vi "Timer IRQ Config Pane.vi"(6 "_SubPanelMessages":refnum<notifier>, 9 "_myEmbeddedToFrameEvent":T7, 10 "_myEmbedded.Exit":refnum<user-event>, 11 "_Property Bundle":cluster{"Name":string, "Value":variant}[](array[cluster])) -> (1 "_Connection Informations":T2, 2 "_Scripter Input":T4)   [LabVIEW 2021]
doc: "Registers analog and digital input interrupts and creates timer interrupts."
uses:
  <vilib>/myRIO/Common/Express VI Framework/typedefs/Config Pane to Framework Ref.ctl
  <vilib>/myRIO/Common/Express VI Framework/typedefs/Data Validate Ref.ctl
  <vilib>/myRIO/Common/Express VI Framework/typedefs/Sub Panel Messages.ctl
  <vilib>/myRIO/Common/Express VI Framework/typedefs/Instrument Driver Method Descriptor Array.ctl
  <vilib>/myRIO/Common/Express VI Framework/typedefs/Instrument Driver Method Descriptor.ctl
  <vilib>/myRIO/Common/Express VI Framework/typedefs/Scripter Input.ctl
  <vilib>/myRIO/Common/Express VI Framework/typedefs/WireThrough Terminal Names.ctl
  <vilib>/myRIO/Common/Express VI Framework/typedefs/Connection Informations.ctl
  <vilib>/myRIO/Common/Express VI Framework/vis/Express VI Framework Strings Global.vi
  <vilib>/myRIO/Express VI/IRQ/Message Globals.vi
panel:
  out "_create Callback?":bool
  in  "_Create Button":bool
  in  "Callback VI Path:":path
  out "_Warning Icon":picture
  out "_Callback VI Path":string caption="Callback VI:"
  in  "_Open Button":bool
  out "_Interval 2":string
  out "_Interval 1":string
  out "_Timer Preview":T1(graph) caption="Preview:"
  out "_Error Message":string
  in  "_callback":refnum<vi>
  in  "_VI Default Name (Edit and make value default)":string="Timer interrupt"
  in  "_WireThrough Info (Edit and make value default)":T3={"WireThrough Top In"="Ref In", "WireThrough Bottom In"="error in (no error)", "WireThrough Top Out"="Ref Out", "WireThrough Bottom Out"="error out"}
  in  "_Template Array (Edit and make value default)":T5=[{"Function Name"="Create Timer IRQ", "VI Path"=path "<vilib>/myRIO/Instrument Drivers/IRQ/Timer IRQ/vis", "Script"=TRUE, "Inputs"=[{"name"="Timer ID", "value"=variant, "Config Pane Only"=TRUE, "Build Array"=FALSE, "Bundle Cluster"=FALSE, "Show Term"=FALSE, "alias"=[], "Required Input"=FALSE}, {"name"="Interval [us]", "value"=variant, "Config Pane Only"=TRUE, "Build Array"=FALSE, "Bundle Cluster"=FALSE, "Show Term"=FALSE, "alias"=[], "Required Input"=FALSE}, {"name"="Callback VI Reference", "value"=variant, "Config Pane Only"=FALSE, "Build Array"=FALSE, "Bundle Cluster"=FALSE, "Show Term"=TRUE, "alias"=[], "Required Input"=FALSE}], "Outputs"=[], "VI Class"=enum."Open", "Controls Refs[]"=[], "Inline"=FALSE}]
  in  "_Default Alias String":string
  in  "Timer ID:":u8 max=7
  in  "Interval (us):":u32=1000000 min=1
  in  "Name:":string="Timer interrupt" caption="Node name:"
  out "_IRQ Learn More":string="Interrupt triggers every time the specified Interval elapses."
  # "NOTE: Tab Order has been set\nfor this Front Panel.\n\nSee Edit>>Set Tabbing Order...\n\nAll controls that are not visible at \nruntime are excluded from Tabbing order\n\nTo exlude a control from context\nhelp prefix its label text with a '-'"
  # "Trigger point"
  # "Time"
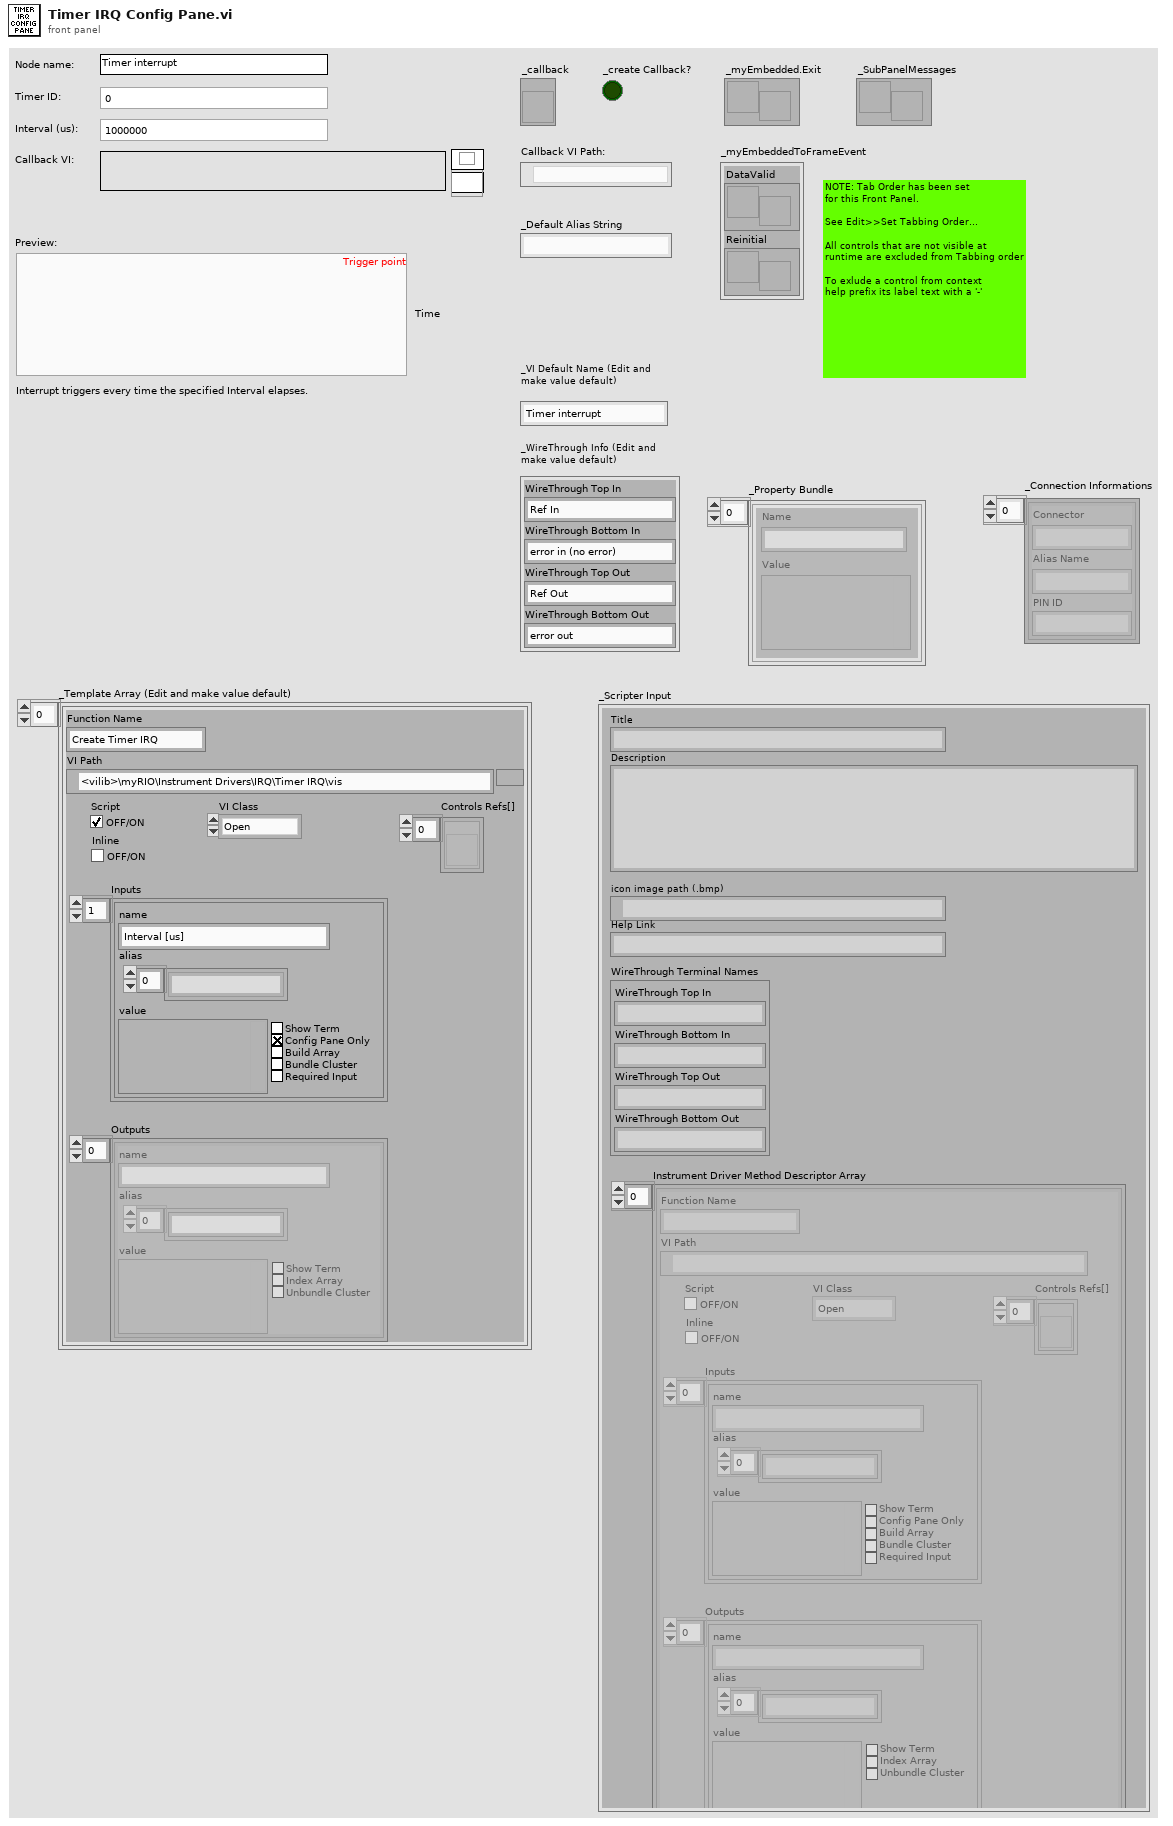
[diagram p1: front panel]
types:
  T1 = cluster{"Analog Preview 3":cluster{"X":sgl, "Y":sgl}[]}[]
  T2 = typedef "Connection Informations.ctl" = cluster{"Connector":string, "Alias Name":string, "PIN ID":string}[]
  T3 = typedef "WireThrough Terminal Names.ctl" = cluster{"WireThrough Top In":string, "WireThrough Bottom In":string, "WireThrough Top Out":string, "WireThrough Bottom Out":string}
  T4 = typedef "Scripter Input.ctl" = cluster{"Title":string, "Description":string, "icon image path (.bmp)":path, "Help Link":string, "WireThrough Terminal Names":T3, "Instrument Driver Method Descriptor Array":T5}
  T5 = typedef "Instrument Driver Method Descriptor Array.ctl" = T6[]
  T6 = typedef "Instrument Driver Method Descriptor.ctl" = cluster{"Function Name":string, "VI Path":path, "Script":bool, "Inputs":cluster{"name":string, "value":variant, "Config Pane Only":bool, "Build Array":bool, "Bundle Cluster":bool, "Show Term":bool, "alias":string[], "Required Input":bool}[], "Outputs":cluster{"name":string, "value":variant, "Show Term":bool, "Index Array":bool, "Unbundle Cluster":bool, "alias":string[]}[], "VI Class":enum16{"Open", "Configure", "Data", "Manage", "Close"}, "Controls Refs[]":refnum<vi>[], "Inline":bool}
  T7 = typedef "Config Pane to Framework Ref.ctl" = cluster{"DataValid":T8, "Reinitial":refnum<user-event>}
  T8 = typedef "Data Validate Ref.ctl" = refnum<user-event>
  T9 = typedef "Sub Panel Messages.ctl" = enum16{"Initialized"}
  T10 = cluster{"left":i16, "top":i16, "right":i16, "bottom":i16}
  T11 = cluster{"name":string, "value":variant, "Config Pane Only":bool, "Build Array":bool, "Bundle Cluster":bool, "Show Term":bool, "alias":string[], "Required Input":bool}[]
  T12 = cluster{"name":string, "value":variant, "Config Pane Only":bool, "Build Array":bool, "Bundle Cluster":bool, "Show Term":bool, "alias":string[], "Required Input":bool}
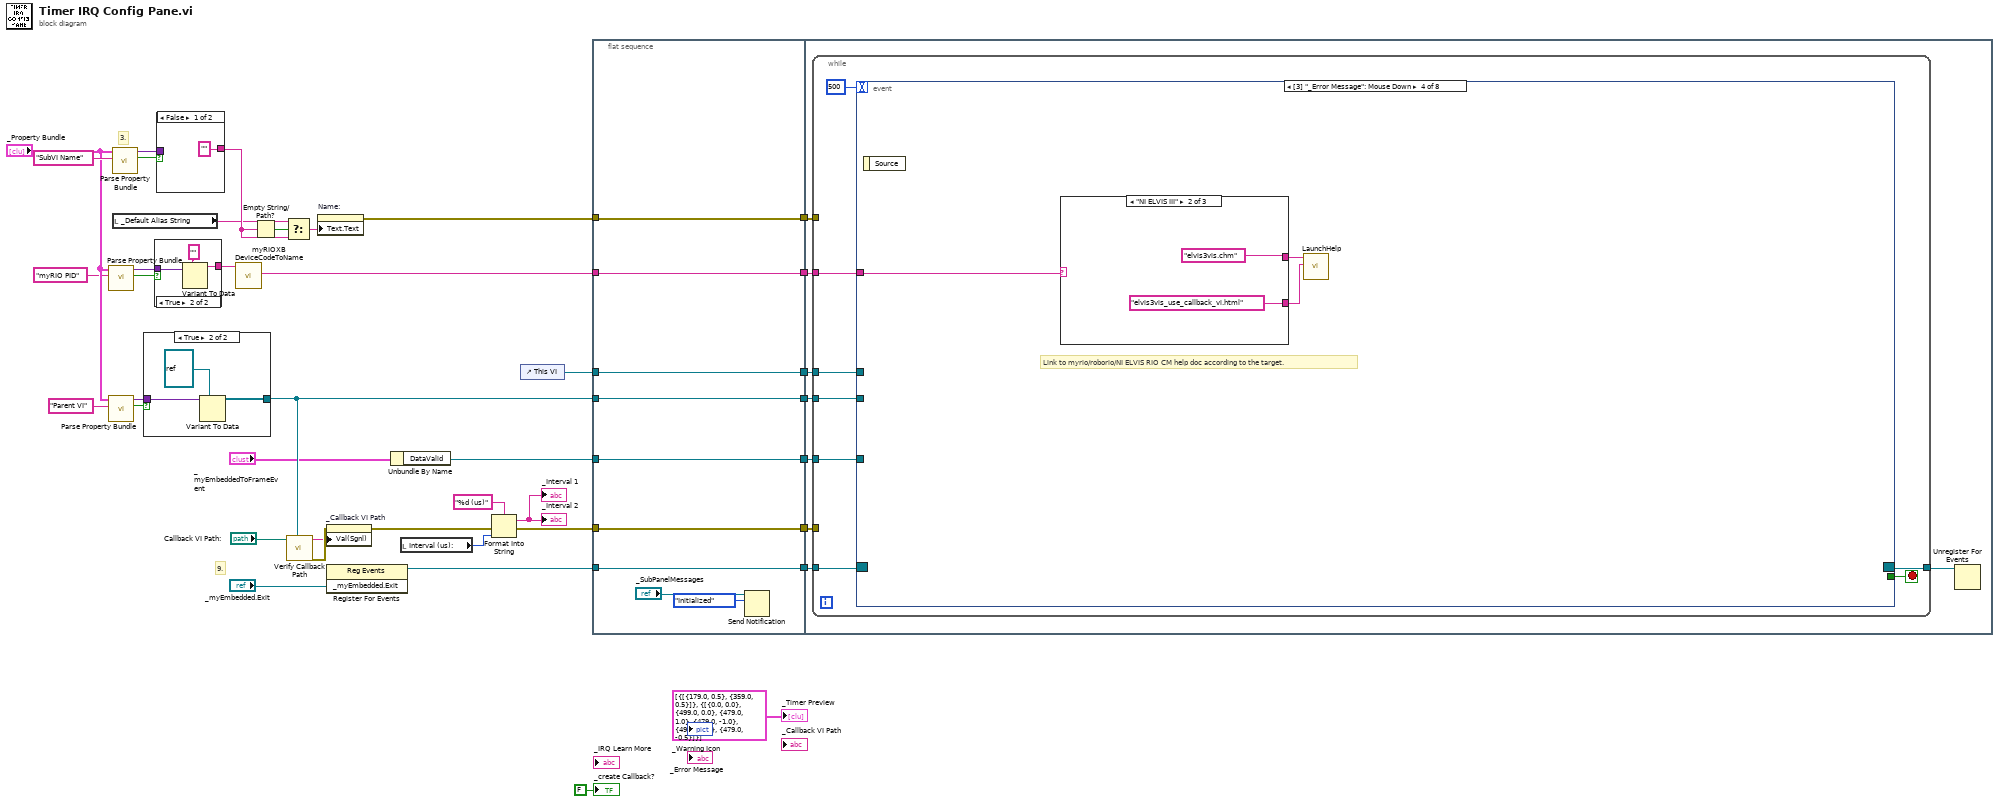
[diagram p0: block diagram]
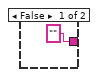
[diagram p2: hidden frame]
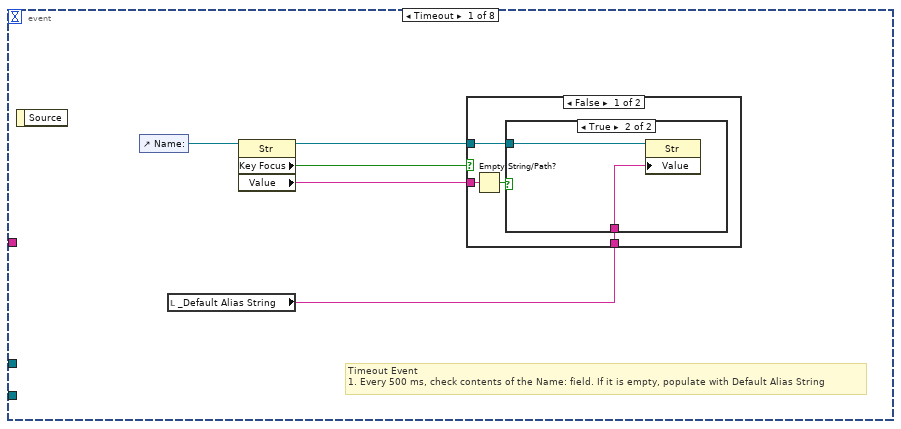
[diagram p3: hidden frame]
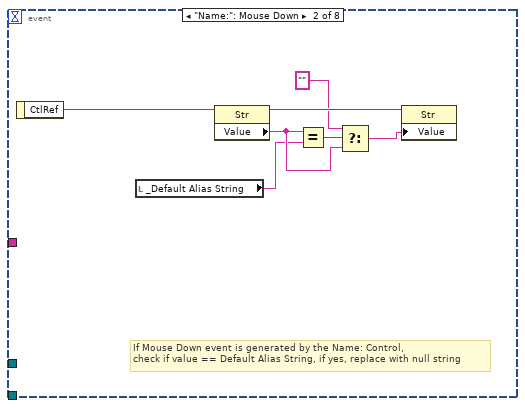
[diagram p6: hidden frame]
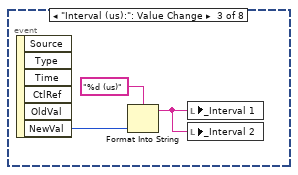
[diagram p7: hidden frame]
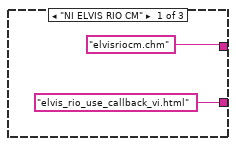
[diagram p8: hidden frame]
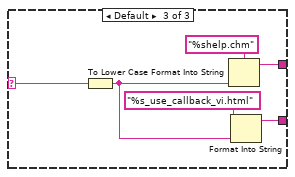
[diagram p9: hidden frame]
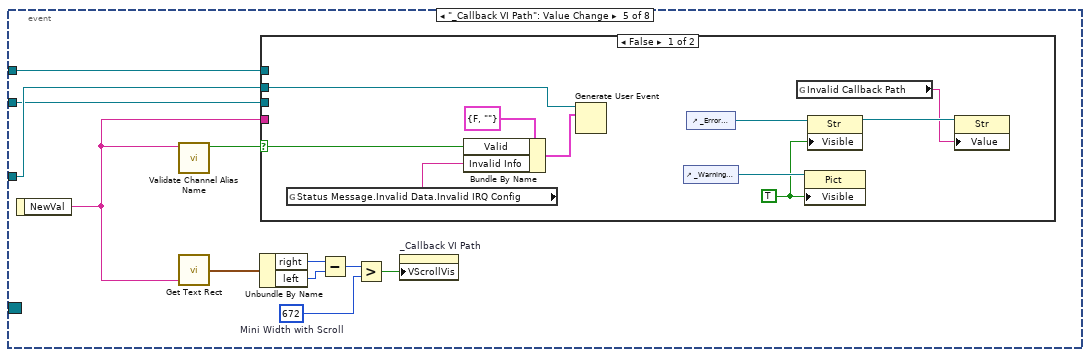
[diagram p10: hidden frame]
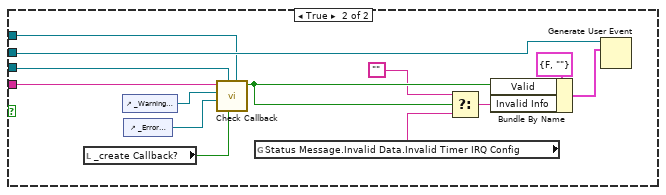
[diagram p11: hidden frame]
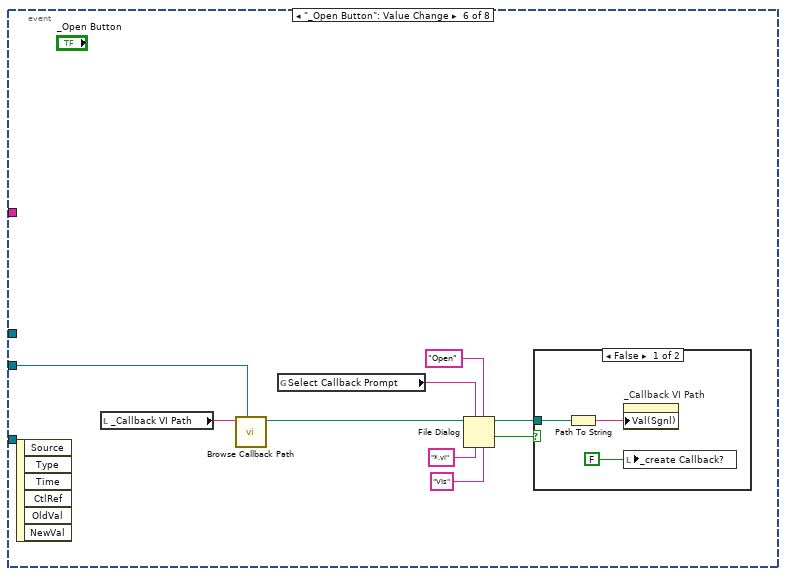
[diagram p12: hidden frame]
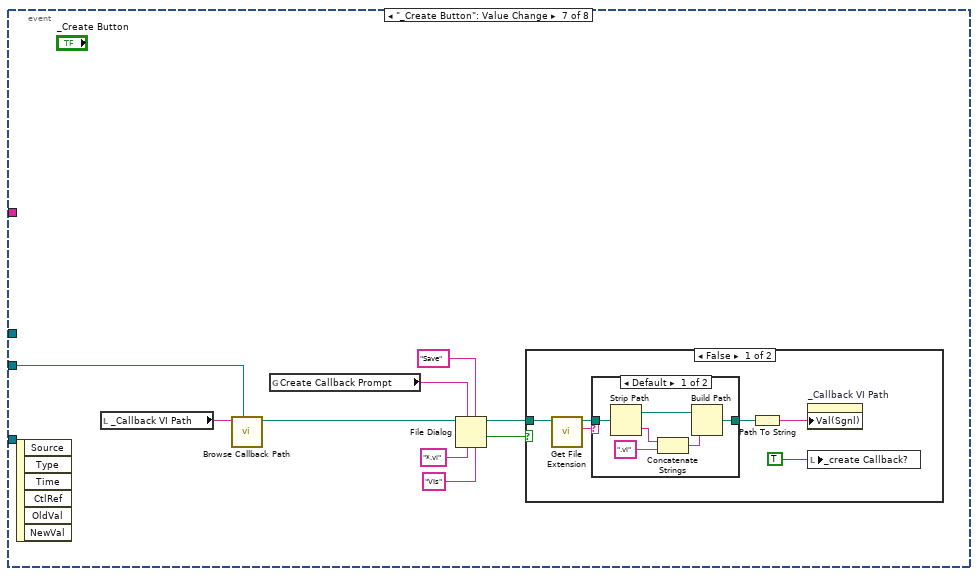
[diagram p14: hidden frame]
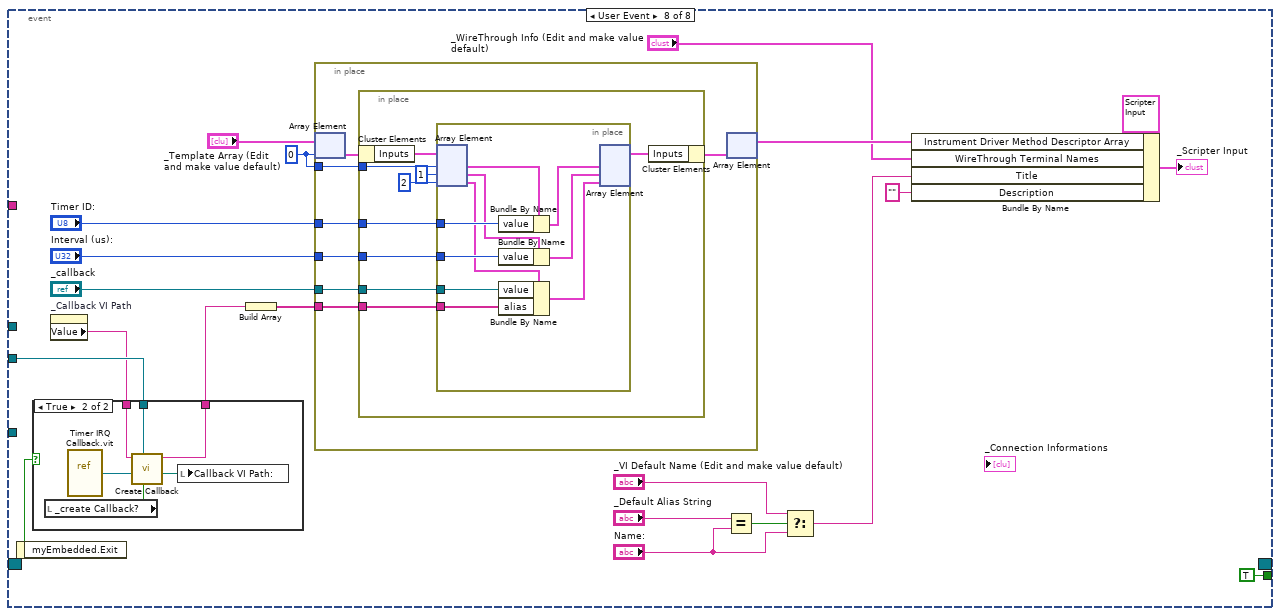
[diagram p17: hidden frame]
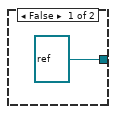
[diagram p19: hidden frame]
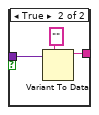
[diagram p20: hidden frame]
diagram:
  # "9."
  # "3."
  n1 = call <vilib>:"Parse Property Bundle.vi"("Name"="myRIO PID", "Property Bundle"="_Property Bundle") -> ("Found?"=w4:bool, "Value"=w5:variant)  [unwired: 8 in]
  n2 = call <vilib>:"Parse Property Bundle.vi"("Name"="Parent VI", "Property Bundle"="_Property Bundle") -> ("Found?"=w28:bool, "Value"=w29:variant)  [unwired: 8 in]
  n3 = call <vilib>:"Parse Property Bundle.vi"("Name"="SubVI Name", "Property Bundle"="_Property Bundle") -> ("Found?"=w37:bool, "Value"=w36:variant)  [unwired: 8 in]
  n4 = local read "_Default Alias String"() -> (w32:string)
  n5 = case shown="True" w28 {
    tunnel: w29 -> [_ w44]
    tunnel: [refnum<vi> refnum ("reference out") w42] -> w20
    frame False {
    }
    frame True {
      n6 = Variant To Data(type=refnum<vi> refnum ("reference out"), Variant=w44) -> (data=w42:refnum<vi>)  [unwired: 1 in, 1 out]
    }
  }
  n7 = case shown="True" w4 {
    tunnel: w5 -> [_ w48]
    tunnel: ["" ("Name") w46] -> w1
    frame False {
    }
    frame True {
      n8 = Variant To Data(type="" ("Name"), Variant=w48) -> (data=w46:string)  [unwired: 1 in, 1 out]
    }
  }
  n9 = case shown="False" w37 {
    tunnel: w36 -> [_ w52]
    tunnel: ["" ("Name") w50] -> w35
    frame False {
    }
    frame True {
      n10 = Variant To Data(type="" ("Name"), Variant=w52) -> (data=w50:string)  [unwired: 1 in, 1 out]
    }
  }
  n11 = call <vilib>:"myRIOXB DeviceCodeToName.vi"("Device Code"=w1) -> ("Name"=w2:string)  [unwired: 10 in]
  n12 = Empty String/Path?(string/path=w35) -> (empty?=w39:bool)
  n13 = Select(t=w32, s=w39, f=w35) -> (s? t:f=w31:string)
  n14 = call <vilib>:"Verify Callback Path.vi"("Parent VI Ref"=w20, "Saved Callback Path"="Callback VI Path:") -> ("error out"=w23:errorcluster, "Valid Path out"=w21:string)  [unwired: 8 in]
  n15 = property on="Name:" class="Str"("Text.Text"=w31) -> (error out=w33:errorcluster)  [unwired: 2 in, 1 out]
  n16 = property on="_Callback VI Path" class="Str"(error in=w23, "Val(Sgnl)"=w21) -> (error out=w22:errorcluster)  [unwired: 1 in, 1 out]
  n17 = register-events("_myEmbedded.Exit") -> (reference out=w34:refnum<event-registration>)  [unwired: 2 in, 1 out]
  n18 = Unbundle By Name("_myEmbeddedToFrameEvent") -> ("DataValid"=w15:T8)
  n19 = local read "Interval (us):"() -> (w25:u32)
  n20 = Format Into String(format string="%d (us)", error in=w22, w25) -> (resulting string=→"_Interval 1" →"_Interval 2":string, error out=w17:errorcluster)  [unwired: 1 in]
  n21 = control-ref of="This VI"() -> (w19:refnum<vi>)
  n22 = flat-sequence {
    tunnel: w15 -> [w56]
    tunnel: w17 -> [w57]
    tunnel: w19 -> [w58]
    tunnel: w20 -> [w59]
    tunnel: w33 -> [w60]
    tunnel: w34 -> [w61]
    tunnel: [w61] -> w14
    tunnel: [w60] -> w13
    tunnel: [w59] -> w12
    tunnel: [w58] -> w11
    tunnel: [w57] -> w10
    tunnel: [w56] -> w9
    tunnel: [w53] -> w3
    tunnel: w2 -> [w53]
    tunnel: w14 -> [w69]
    tunnel: w13 -> [w67]
    tunnel: w12 -> [w66]
    tunnel: w11 -> [w65]
    tunnel: w10 -> [w64]
    tunnel: w9 -> [w63]
    tunnel: w3 -> [w62]
    frame #0 {
      n23 = Send Notification(notification=Sub_Panel_Messages."Initialized", notifier="_SubPanelMessages") -> ()  [unwired: 1 in, 2 out]
    }
    frame #1 {
      n24 = while {
        tunnel: w69 -> [w76]
        tunnel: w63 -> [w73]
        tunnel: [w74] -> w68
        tunnel: w67 -> [_]
        tunnel: w66 -> [w72]
        tunnel: w65 -> [w71]
        tunnel: w64 -> [_]
        tunnel: w62 -> [w70]
        stop <- w75 stop-if-true
        n25 = event shown="[3] \"_Error Message\": Mouse Down" {
          selector: w76 -> [_ _ _ _ _ _ _ _]
          dyn-events: [_ _ _ _ _ _ _ _] -> w74
          timeout: 500 -> [_ _ _ _ _ _ _ _]
          tunnel: [_ _ _ _ _ _ _ TRUE ("Valid Callback?")] -> w75
          tunnel: w73 -> [_ _ _ _ w122 _ _ _]
          tunnel: w72 -> [_ _ _ _ w121 w147 w158 w184]
          tunnel: w71 -> [_ _ _ _ w120 _ _ _]
          tunnel: w70 -> [_ _ _ w99 _ _ _ _]
          event Timeout {
            # "Timeout Event\n1. Every 500 ms, check contents of the Name: field. If it is empty, populate with Default Alias String"
            n26 = event-data() -> ()  [unwired: 1 in, 1 out]
            n27 = control-ref of="Name:"() -> (w79:refnum<vi>)
            n28 = local read "_Default Alias String"() -> (w78:string)
            n29 = property on="Property Node" class="Str"(reference=w79) -> (reference out=w82:refnum<vi>, "Key Focus"=w81:bool, "Value"=w80:string)  [unwired: 1 in, 1 out]
            n30 = case shown="False" w81 {
              tunnel: w80 -> [w86 _]
              tunnel: w82 -> [w84 _]
              tunnel: w78 -> [w83 _]
              frame False {
                n31 = Empty String/Path?(string/path=w86) -> (empty?=w85:bool)
                n32 = case shown="True" w85 {
                  tunnel: w84 -> [_ w88]
                  tunnel: w83 -> [_ w87]
                  frame False {
                  }
                  frame True {
                    n33 = property on="Property Node" class="Str"(reference=w88, "Value"=w87) -> ()  [unwired: 1 in, 2 out]
                  }
                }
              }
              frame True {
              }
            }
          }
          event "Name:": Mouse Down {
            # "If Mouse Down event is generated by the Name: Control,\ncheck if value == Default Alias String, if yes, replace with null string"
            n34 = event-data() -> ("CtlRef"=w90:refnum<vi>)  [unwired: 1 in]
            n35 = local read "_Default Alias String"() -> (w89:string)
            n36 = property class="Str"(reference=w90) -> (reference out=w94:refnum<vi>, "Value"=w95:string)  [unwired: 1 in, 1 out]
            n37 = Equal?(x=w95, y=w89) -> (x = y?=w91:bool)
            n38 = Select(t="", s=w91, f=w95) -> (s? t:f=w93:string)
            n39 = property class="Str"(reference=w94, "Value"=w93) -> ()  [unwired: 1 in, 2 out]
          }
          event "Interval (us):": Value Change {
            n40 = event-data() -> ("NewVal"=w98:u32)  [unwired: 1 in, 5 out]
            n41 = Format Into String(format string="%d (us)", w98) -> (resulting string=w96:string)  [unwired: 2 in, 1 out]
            n42 = local write "_Interval 1"(w96) -> ()
            n43 = local write "_Interval 2"(w96) -> ()
          }
          event "_Error Message": Mouse Down {
            # "Link to myrio/roborio/NI ELVIS RIO CM help doc according to the target."
            n44 = event-data() -> ()  [unwired: 1 in, 1 out]
            n45 = case shown="\"NI ELVIS III\"" w99 {
              selector: w99 -> [_ _ w106]
              tunnel: ["elvisriocm.chm" ("Help File") "elvis3vis.chm" ("Help File") w108] -> w101
              tunnel: ["elvis_rio_use_callback_vi.html" ("Help Topic") "elvis3vis_use_callback_vi.html" ("Help Topic") w107] -> w100
              frame "NI ELVIS RIO CM" {
              }
              frame "NI ELVIS III" {
              }
              frame Default {
                n46 = To Lower Case(string=w106) -> (all lower case string=w110:string)
                n47 = Format Into String(format string="%shelp.chm" ("Help File"), w110) -> (resulting string=w108:string)  [unwired: 2 in, 1 out]
                n48 = Format Into String(format string="%s_use_callback_vi.html" ("Help Topic"), w110) -> (resulting string=w107:string)  [unwired: 2 in, 1 out]
              }
            }
            n49 = call <vilib>:"LaunchHelp.vi"("Help Topic"=w100, "Help File"=w101) -> ()  [unwired: 10 in]
          }
          event "_Callback VI Path": Value Change {
            w115 = i16 672  # Mini Width with Scroll
            n50 = event-data() -> ("NewVal"=w112:string)  [unwired: 1 in]
            n51 = call <vilib>:"Validate Channel Alias Name.vi"("Channel Alias"=w112) -> ("Valid?"=w113:bool)  [unwired: 9 in, 1 out]
            n52 = call <vilib>:"Get Text Rect.vi"("text"=w112) -> ("rect"=w119:T10)  [unwired: 8 in]
            n53 = Unbundle By Name(w119) -> ("right"=w118:i16, "left"=w117:i16)
            n54 = case shown="False" w113 {
              selector: w113 -> [w129 _]
              tunnel: w122 -> [w130 w145]
              tunnel: w121 -> [_ w144]
              tunnel: w120 -> [_ w141]
              tunnel: w112 -> [_ w140]
              frame False {
                w126 = TRUE ("Visible")
                n55 = global read "Express VI Framework Strings Global.vi" "Status Message.Invalid Data.Invalid IRQ Config"() -> (w125:string)
                n56 = Bundle By Name(cluster=cluster{"Valid":bool, "Invalid Info":string} {"Valid"=FALSE, "Invalid Info"=""} ("event data"), "Valid"=w129, "Invalid Info"=w125) -> (w131:cluster{"Valid":bool, "Invalid Info":string})
                n57 = Generate User Event(user event=w130, event data cluster=w131) -> ()  [unwired: 2 in, 2 out]
                n58 = control-ref of="_Warning Icon"() -> (w127:refnum<vi>)
                n59 = control-ref of="_Error Message"() -> (w128:refnum<vi>)
                n60 = global read "Message Globals.vi" "Invalid Callback Path"() -> (w123:string)
                n61 = property class="Pict"(reference=w127, "Visible"=w126) -> ()  [unwired: 1 in, 2 out]
                n62 = property class="Str"(reference=w128, "Visible"=w126) -> (reference out=w124:refnum<vi>)  [unwired: 1 in, 1 out]
                n63 = property class="Str"(reference=w124, "Value"=w123) -> ()  [unwired: 1 in, 2 out]
              }
              frame True {
                n64 = local read "_create Callback?"() -> (w139:bool)
                n65 = control-ref of="_Warning Icon"() -> (w142:refnum<vi>)
                n66 = control-ref of="_Error Message"() -> (w143:refnum<vi>)
                n67 = call <vilib>:"Check Callback.vi"("Config VI Ref"=w141, "Create Callback?"=w139, "Parent VI Ref"=w144, "Error Message Ref"=w143, "Warning Icon Ref"=w142, "Callback Path"=w140) -> ("Valid Callback?"=w136:bool)  [unwired: 5 in]
                n68 = global read "Express VI Framework Strings Global.vi" "Status Message.Invalid Data.Invalid Timer IRQ Config"() -> (w134:string)
                n69 = Select(t="", s=w136, f=w134) -> (s? t:f=w133:string)
                n70 = Bundle By Name(cluster=cluster{"Valid":bool, "Invalid Info":string} {"Valid"=FALSE, "Invalid Info"=""} ("event data"), "Valid"=w136, "Invalid Info"=w133) -> (w137:cluster{"Valid":bool, "Invalid Info":string})
                n71 = Generate User Event(user event=w145, event data cluster=w137) -> ()  [unwired: 2 in, 2 out]
              }
            }
            n72 = Subtract(x=w118, y=w117) -> (x-y=w116:i16)
            n73 = Greater?(x=w116, y=w115) -> (0:w114:bool)
            n74 = property on="_Callback VI Path" class="Str"("VScrollVis"=w114) -> ()  [unwired: 2 in, 2 out]
          }
          event "_Open Button": Value Change {
            n75 = event-data() -> ()  [unwired: 1 in, 6 out]
            n76 = local read "_Callback VI Path"() -> (w148:string)
            n77 = call <vilib>:"Browse Callback Path.vi"("Parent VI Ref"=w147, "Init Path in"=w148) -> ("Init Path out"=w146:path)  [unwired: 9 in]
            n78 = global read "Message Globals.vi" "Select Callback Prompt"() -> (w150:string)
            n79 = File Dialog(4:"VIs" ("pattern label"), 5:"Open" ("button label"), 6:"*.vi" ("pattern (all files)"), 7:w150, 11:w146) -> (1:w153:bool, 3:w154:path)  [unwired: 2 in, 2 out]
            n80 = case shown="False" w153 {
              tunnel: w154 -> [w157 _]
              frame False {
                n81 = Path To String(path=w157) -> (string=w156:string)
                n82 = property on="_Callback VI Path" class="Str"("Val(Sgnl)"=w156) -> ()  [unwired: 2 in, 2 out]
                n83 = local write "_create Callback?"(FALSE ("_create Callback?")) -> ()
              }
              frame True {
              }
            }
          }
          event "_Create Button": Value Change {
            n84 = event-data() -> ()  [unwired: 1 in, 6 out]
            n85 = local read "_Callback VI Path"() -> (w160:string)
            n86 = call <vilib>:"Browse Callback Path.vi"("Parent VI Ref"=w158, "Init Path in"=w160) -> ("Init Path out"=w159:path)  [unwired: 9 in]
            n87 = global read "Message Globals.vi" "Create Callback Prompt"() -> (w162:string)
            n88 = File Dialog(4:"VIs" ("pattern label"), 5:"Save" ("button label"), 6:"*.vi" ("pattern (all files)"), 7:w162, 11:w159) -> (1:w165:bool, 3:w166:path)  [unwired: 2 in, 2 out]
            n89 = case shown="False" w165 {
              tunnel: w166 -> [w168 _]
              frame False {
                n90 = call <vilib>:"Get File Extension.vi"("file"=w168) -> ("lowercase file extension"=w169:string, "dup file"=w170:path)  [unwired: 6 in, 3 out]
                n91 = case shown="Default" w169 {
                  tunnel: w170 -> [w178 w179]
                  tunnel: [w174 w179] -> w167
                  frame Default {
                    n92 = Strip Path(path=w178) -> (stripped path=w177:path, name=w176:string)
                    n93 = Concatenate Strings(w176, ".vi" ("string")) -> (w175:string)
                    n94 = Build Path(base path=w177, name or relative path=w175) -> (appended path=w174:path)
                  }
                  frame "vi" {
                  }
                }
                n95 = Path To String(path=w167) -> (string=w172:string)
                n96 = property on="_Callback VI Path" class="Str"("Val(Sgnl)"=w172) -> ()  [unwired: 2 in, 2 out]
                n97 = local write "_create Callback?"(TRUE ("_create Callback?")) -> ()
              }
              frame True {
              }
            }
          }
          event User Event {
            w187 = 0
            n98 = event-data() -> ("myEmbedded.Exit"=w180:bool)  [unwired: 1 in]
            n99 = property on="_Callback VI Path" class="Str"() -> ("Value"=w181:string)  [unwired: 2 in, 2 out]
            n100 = case shown="True" w180 {
              tunnel: w184 -> [_ w207]
              tunnel: [w201 w205] -> w182
              tunnel: w181 -> [w201 w204]
              frame False {
              }
              frame True {
                n101 = local read "_create Callback?"() -> (w203:bool)
                n102 = vi-ref <vilib>:"Timer IRQ Callback.vit"() -> (w202:refnum<vi>)
                n103 = call <vilib>:"Create Callback.vi"("Create Callback?"=w203, "Parent VI Ref"=w207, "Template VI Ref"=w202, "Callback Path"=w204) -> ("Saved Callback Path"=w206:path, "Dup Callback Path"=w205:string)  [unwired: 6 in]
                n104 = local write "Callback VI Path:"(w206) -> ()
              }
            }
            n105 = Build Array(w182) -> (w186:string[])
            n106 = in-place {
              in-place-border: "Timer ID:" -> [w213]
              in-place-border: "Interval (us):" -> [w212]
              in-place-border: "_callback" -> [w211]
              in-place-border: w187 -> [w209]
              in-place-border: w186 -> [w208]
              n107 = in-place-array #1("_Template Array (Edit and make value default)", w187) -> (w214:T6)
              n108 = in-place {
                in-place-border: w213 -> [w222]
                in-place-border: w212 -> [w221]
                in-place-border: w211 -> [w220]
                in-place-border: w209 -> [w215]
                in-place-border: w208 -> [w216]
                n109 = in-place-cluster #2(w214) -> ("Inputs"=w223:T11)
                n110 = in-place {
                  in-place-border: w222 -> [w232]
                  in-place-border: w221 -> [w231]
                  in-place-border: w220 -> [w230]
                  in-place-border: w216 -> [w228]
                  n111 = in-place-array #3(w223, w215, 1, 2) -> (w233:T12, w227:T12, w226:T12)
                  n112 = Bundle By Name(cluster=w233, "value"=w232) -> (w229:T12)
                  n113 = Bundle By Name(cluster=w227, "value"=w231) -> (w225:T12)
                  n114 = Bundle By Name(cluster=w226, "value"=w230, "alias"=w228) -> (w224:T12)
                  n115 = in-place-array #3(w229, w225, w224) -> (w219:T11)  [unwired: 3 out]
                }
                n116 = in-place-cluster #2("Inputs"=w219) -> (w210:T6)
              }
              n117 = in-place-array #1(w210) -> (w193:T5)  [unwired: 1 out]
            }
            n118 = Equal?(x="_Default Alias String", y="Name:") -> (x = y?=w196:bool)
            n119 = Select(t="_VI Default Name (Edit and make value default)", s=w196, f="Name:") -> (s? t:f=w197:string)
            n120 = Bundle By Name(cluster=T4 {"Title"="", "Description"="", "icon image path (.bmp)"=path "", "Help Link"="", "WireThrough Terminal Names"={"WireThrough Top In"="", "WireThrough Bottom In"="", "WireThrough Top Out"="", "WireThrough Bottom Out"=""}, "Instrument Driver Method Descriptor Array"=[]} ("Scripter Input"), "Instrument Driver Method Descriptor Array"=w193, "WireThrough Terminal Names"="_WireThrough Info (Edit and make value default)", "Title"=w197, "Description"="" ("Title")) -> (→"_Scripter Input":T4)
          }
        }
      }
      n121 = Unregister For Events(event registration refnum=w68) -> ()  [unwired: 1 in, 1 out]
    }
  }
  "_Timer Preview" <- T1 [{"Analog Preview 3"=[{"X"=179.0, "Y"=0.5}, {"X"=359.0, "Y"=0.5}]}, {"Analog Preview 3"=[{"X"=0.0, "Y"=0.0}, {"X"=499.0, "Y"=0.0}, {"X"=479.0, "Y"=1.0}, {"X"=479.0, "Y"=-1.0}, {"X"=499.0, "Y"=0.0}, {"X"=479.0, "Y"=-0.5}]}] ("Timer Preview")
  "_create Callback?" <- FALSE ("_create Callback?")
